vi "read.vi"(8 "error in (no error)":errorcluster, 10 "block size":i32, 11 "SignalReader in":refnum<class "SignalReaderDL091205FPGA.lvclass">) -> (0 "error out":errorcluster, 1 "finished?":bool, 2 "signals read":dbl[][](graph), 3 "SignalReader out":refnum<class "SignalReaderDL091205FPGA.lvclass">, 4 "buffer overflow?":bool)   [LabVIEW 2010, in "SignalReaderDL091205FPGA.lvclass"]
uses:
  SignalReaderDL091205FPGA.lvclass
  SignalReaderDL091205FPGA.lvclass/SignalReaderDL091205FPGA.ctl
  FPGAWrapper/GenericFPGAWrapper/GenericFPGAWrapper/GenericFPGAWrapper.lvclass
  GenericSignalReader/GenericSignalReader/GenericSignalReader.lvclass
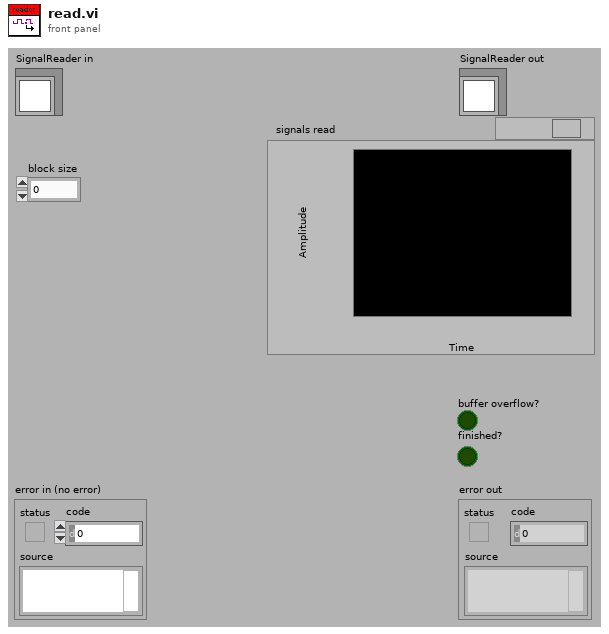
[diagram p1: front panel]
types:
  T1 = typedef "pixel_raw_data_array.ctl" = dbl[][]
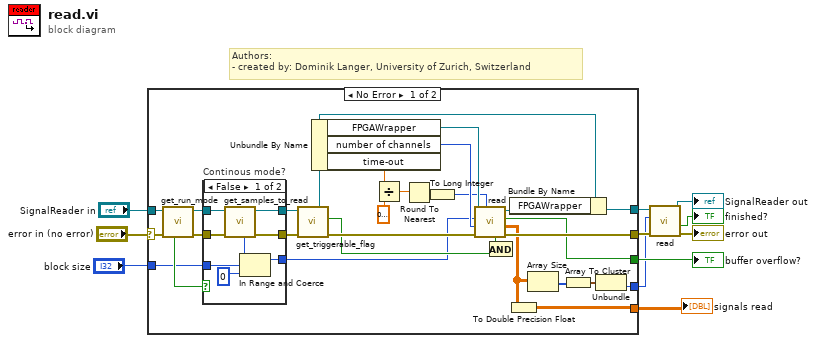
[diagram p0: block diagram]
diagram:
  # "Authors: \n- created by: Dominik Langer, University of Zurich, Switzerland"
  n1 = case shown="No Error" "error in (no error)" {
    selector: "error in (no error)" -> [w25 w51]
    tunnel: "SignalReader in" -> [w24 w52]
    tunnel: [w37 w52] -> w5
    tunnel: [w36 w51] -> w7
    tunnel: "block size" -> [w23 _]
    tunnel: [w35 _] -> w1
    tunnel: [w34 _] -> w8
    tunnel: [w19 _] -> w2
    frame No Error {
      n2 = call-dynamic "get_run_mode.vi"("error in (no error)"=w25, "GenericPlugin in"=w24) -> ("error out"=w26:errorcluster, "GenericPlugin out"=w27:refnum<class "SignalReaderDL091205FPGA.lvclass">, "is free run?"=w28:bool)  [unwired: 5 in, 2 out]
      n3 = case "Continous mode?" shown="False" w28 {
        tunnel: [w47 w48] -> w17
        tunnel: [w45 w49] -> w16
        tunnel: w23 -> [w43 w50]
        tunnel: [w42 w50] -> w12
        tunnel: w26 -> [w41 w48]
        tunnel: w27 -> [w40 w49]
        frame False {
          n4 = call-dynamic "get_samples_to_read.vi"("error in (no error)"=w41, "GenericSignalReader in"=w40) -> ("error out"=w47:errorcluster, "GenericSignalReader out"=w45:refnum<class "SignalReaderDL091205FPGA.lvclass">, "samples still to be read"=w44:i32)  [unwired: 5 in, 2 out]
          n5 = In Range and Coerce(upper limit=w44, x=w43, lower limit=0) -> (coerced(x)=w42:i32)  [unwired: 1 out]
        }
        frame True {
        }
      }
      n6 = call-dynamic "get_triggerable_flag.vi"("error in (no error)"=w17, "GenericSignalReader in"=w16) -> ("error out"=w18:errorcluster, "triggerable?"=w14:bool)  [unwired: 7 in, 1 out]
      n7 = Unbundle By Name(w16) -> ("FPGAWrapper"=w39:refnum<class "GenericFPGAWrapper.lvclass">, "number of channels"=w33:i32, "time-out"=w32:dbl[unit])
      n8 = Divide(x=w32, y=dbl[unit] 0.001) -> (x/y=w30:dbl)
      n9 = Round To Nearest(number=w30) -> (nearest integer value=w29:dbl)
      n10 = To Long Integer(number=w29) -> (32bit integer=w15:i32)
      n11 = call-dynamic "read.vi"("timeout (ms)"=w15, "error in (no error)"=w18, "number of channels"=w33, "block size"=w12, "GenericFPGAWrapper in"=w39) -> ("error out"=w36:errorcluster, "channels raw data block"=w20:T1, "FIFO full?"=w34:bool, "GenericFPGAWrapper out"=w38:refnum<class "GenericFPGAWrapper.lvclass">, "timed out?"=w13:bool)  [unwired: 2 out]
      n12 = And(x=w13, y=w14) -> ()  [unwired: 1 out]
      n13 = To Double Precision Float(number=w20) -> (double precision float=w35:T1)
      n14 = Bundle By Name(cluster=w16, "FPGAWrapper"=w38) -> (w37:refnum<class "SignalReaderDL091205FPGA.lvclass">)
      n15 = Array Size(array=w20) -> (size(s)=w21:i32[])
      n16 = Array To Cluster(array=w21) -> (cluster=w22:cluster{"[0]":i32, "[1]":i32})
      n17 = Unbundle(w22) -> ("[1]"=w19:i32)  [unwired: 1 out]
    }
    frame Error {
    }
  }
  "buffer overflow?" <- w8
  "signals read" <- w1
  n18 = call-parent "read.vi"("error in (no error)"=w7, "block size"=w2, "SignalReader in"=w5) -> ("error out"=→"error out":errorcluster, "finished?"=→"finished?":bool, "SignalReader out"=→"SignalReader out":refnum<class "SignalReaderDL091205FPGA.lvclass">)  [unwired: 4 in, 2 out]
